vi "SetCodePreferences.vi"(10 "Color choices":T1={"Quote"=46086, "Comment"=15665920, "Python"=14453248, "Text"=0, "Triple Quote"=9306312, "function"=239, "Line numbers"=9306312, "REPL Err"=15665920, "REPL Text"=0, "Text Bkgd"=16777215, "REPL Bkgd"=16777215}, 11 "PrefFile":string="Colors.txt") -> ()   [LabVIEW 2020]
uses:
  ColorText/ColorGlobals.vi
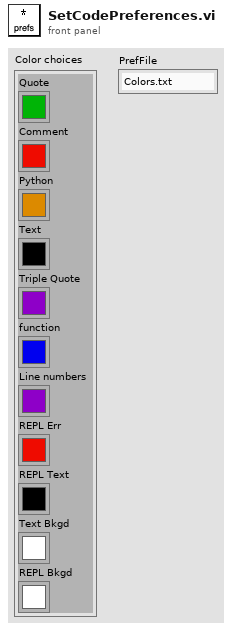
[diagram p1: front panel]
types:
  T1 = cluster{"Quote":u32, "Comment":u32, "Python":u32, "Text":u32, "Triple Quote":u32, "function":u32, "Line numbers":u32, "REPL Err":u32, "REPL Text":u32, "Text Bkgd":u32, "REPL Bkgd":u32}
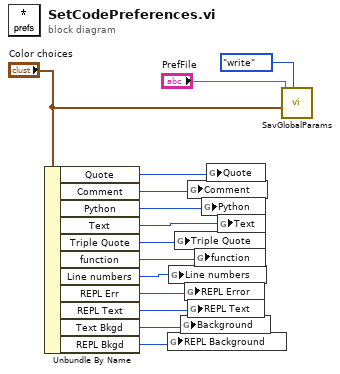
[diagram p0: block diagram]
diagram:
  n1 = Unbundle By Name("Color choices") -> ("Quote"=w14:u32, "Comment"=w13:u32, "Python"=w12:u32, "Text"=w11:u32, "Triple Quote"=w10:u32, "function"=w9:u32, "Line numbers"=w6:u32, "REPL Err"=w7:u32, "REPL Text"=w8:u32, "Text Bkgd"=w5:u32, "REPL Bkgd"=w4:u32)
  n2 = global write "ColorGlobals.vi" "REPL Background"(w4) -> ()
  n3 = global write "ColorGlobals.vi" "Line numbers"(w6) -> ()
  n4 = global write "ColorGlobals.vi" "Triple Quote"(w10) -> ()
  n5 = global write "ColorGlobals.vi" "Background"(w5) -> ()
  n6 = global write "ColorGlobals.vi" "REPL Error"(w7) -> ()
  n7 = global write "ColorGlobals.vi" "Comment"(w13) -> ()
  n8 = global write "ColorGlobals.vi" "REPL Text"(w8) -> ()
  n9 = global write "ColorGlobals.vi" "function"(w9) -> ()
  n10 = global write "ColorGlobals.vi" "Python"(w12) -> ()
  n11 = global write "ColorGlobals.vi" "Quote"(w14) -> ()
  n12 = global write "ColorGlobals.vi" "Text"(w11) -> ()
  n13 = call "SavGlobalParams.vi"("Task"=enum16{"read", "write"}."write", "Color choices"="Color choices", "FileName"="PrefFile") -> ()  [unwired: 8 in, 1 out]
